vi "Read Number of column.vi"(0 "PDF Table Class":refnum<class "Pdfp Table Class.lvclass">, 11 "error in (no error)":errorcluster) -> (4 "PDF Table Class duplicate":refnum<class "Pdfp Table Class.lvclass">, 8 "# columns":i32, 15 "error duplicate":errorcluster)   [LabVIEW 2019, in "Exaprom PDF.lvlib" / "Pdfp Table Class.lvclass"]
doc: "Version 2.0\nDeveloped by Jean-Marc Simard\nCopyright © 2012, Exaprom Inc.\nAll rights reserved.\nLicense: BSD\n\nWith iTextSharp 4.1.6 (http://itextsharp.sourceforge.net)\nunder Mozilla Public License Version 1.1\n(http://www.mozilla.org/MPL/MPL-1.1.html)"
uses:
  Pdfp Table Class.lvclass
  Pdfp Table Class.lvclass/Pdfp Table Class.ctl
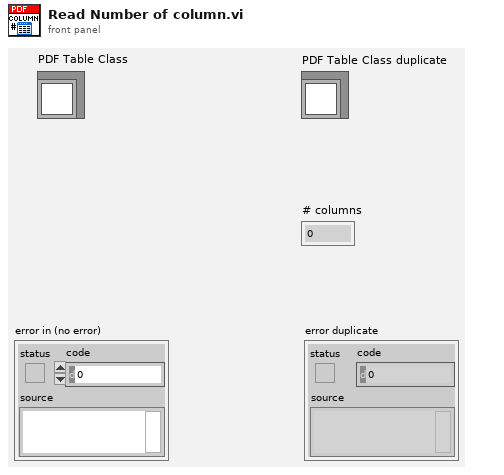
[diagram p1: front panel]
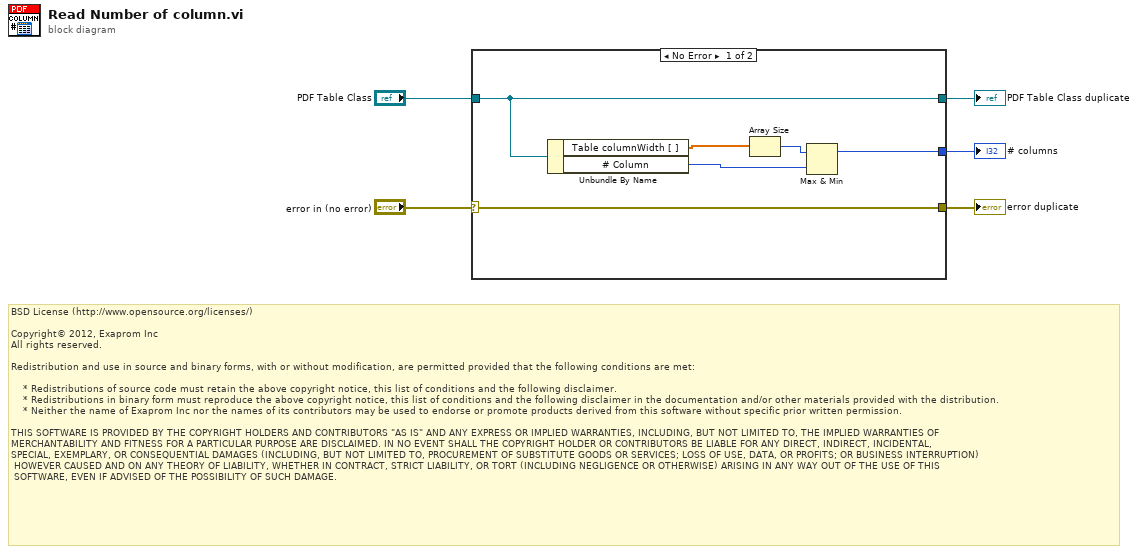
[diagram p0: block diagram]
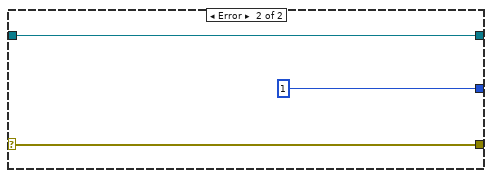
[diagram p2: hidden frame]
diagram:
  # "BSD License (http://www.opensource.org/licenses/)\n\nCopyright© 2012, Exaprom Inc\nAll rights reserved.\n\nRedistribution and use in source and binary forms, with or without modification, are permitted provided that the following conditions are met:\n\n    * Redistributions of source code must retain the above copyright notice, this list of conditions and the following disclaimer.\n    * Redistributions in binary form must reproduce the above copyright notice, this list of conditions and the following disclaimer in the documentation and/or other materials provided with the distribution.\n    * Neither the name of Exaprom Inc nor the names of its contributors may be used to endorse or promote products derived from this software without specific prior written permission.\n\nTHIS SOFTWARE IS PROVIDED BY THE COPYRIGHT HOLDERS AND CONTRIBUTORS \"AS IS\" AND ANY EXPRESS OR IMPLIED WARRANTIES, INCLUDING, BUT NOT LIMITED TO, THE IMPLIED WARRANTIES OF \nMERCHANTABILITY AND FITNESS FOR A PARTICULAR PURPOSE ARE DISCLAIMED. IN NO EVENT SHALL THE COPYRIGHT HOLDER OR CONTRIBUTORS BE LIABLE FOR ANY DIRECT, INDIRECT, INCIDENTAL,\nSPECIAL, EXEMPLARY, OR CONSEQUENTIAL DAMAGES (INCLUDING, BUT NOT LIMITED TO, PROCUREMENT OF SUBSTITUTE GOODS OR SERVICES; LOSS OF USE, DATA, OR PROFITS; OR BUSINESS INTERRUPTION)\n HOWEVER CAUSED AND ON ANY THEORY OF LIABILITY, WHETHER IN CONTRACT, STRICT LIABILITY, OR TORT (INCLUDING NEGLIGENCE OR OTHERWISE) ARISING IN ANY WAY OUT OF THE USE OF THIS\n SOFTWARE, EVEN IF ADVISED OF THE POSSIBILITY OF SUCH DAMAGE."
  n1 = case shown="No Error" "error in (no error)" {
    selector: "error in (no error)" -> [w11 w14]
    tunnel: [w11 w14] -> w5
    tunnel: [w6 1] -> w3
    tunnel: "PDF Table Class" -> [w9 w12]
    tunnel: [w9 w12] -> w1
    frame No Error {
      n2 = Unbundle By Name(w9) -> ("Table columnWidth [ ]"=w8:sgl[], "# Column"=w7:u16)
      n3 = Array Size(array=w8) -> (size(s)=w10:i32)
      n4 = Max & Min(x=w10, y=w7) -> (max(x,y)=w6:i32)  [unwired: 1 out]
    }
    frame Error {
    }
  }
  "error duplicate" <- w5
  "# columns" <- w3
  "PDF Table Class duplicate" <- w1
